vi "Array2GrayPic.vi"(7 "Pic Reference":refnum<vi>, 8 "Threshold (min)":dbl, 9 "Threshold (max)":dbl, 10 "Auto Scale?":bool, 11 "Intensity":dbl[][](array[numeric])) -> (3 "Gray Picture":picture caption="HSV to RGB Picture")   [LabVIEW 2015]
uses:
  <vilib>/picture/picture.llb/Draw True-Color Pixmap.vi
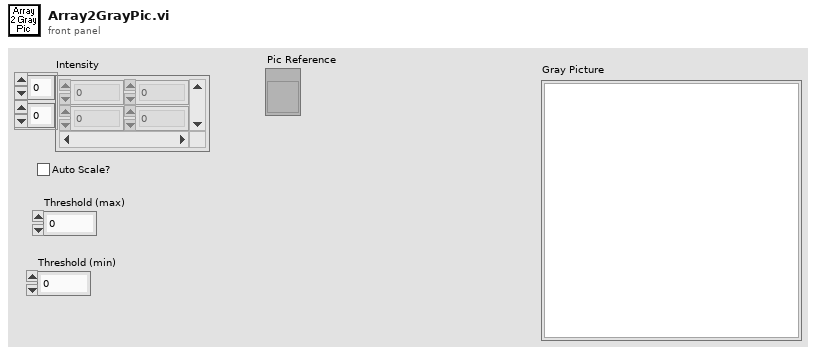
[diagram p1: front panel]
types:
  T1 = typedef "LVBoundsTypeDef.ctl" = cluster{"Width":u32, "Height":u32}
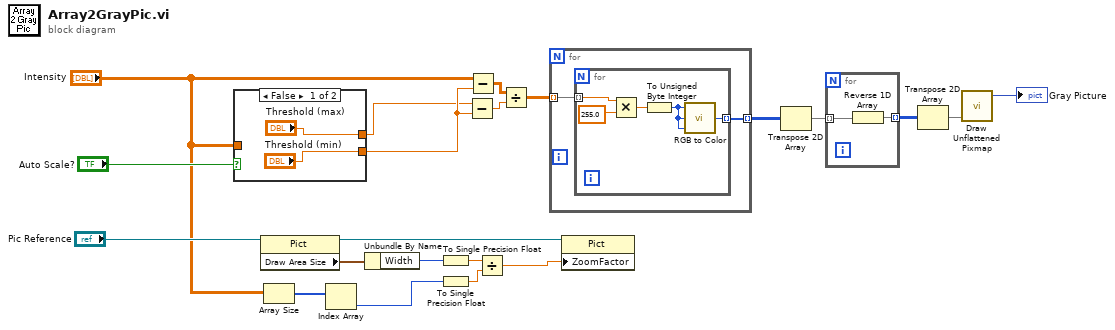
[diagram p0: block diagram]
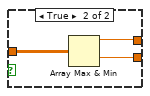
[diagram p2: hidden frame]
diagram:
  n1 = case shown="False" "Auto Scale?" {
    tunnel: "Intensity" -> [_ w26]
    tunnel: ["Threshold (max)" w25] -> w17
    tunnel: ["Threshold (min)" w24] -> w18
    frame False {
    }
    frame True {
      n2 = Array Max & Min(array=w26) -> (max value=w25:dbl, min value=w24:dbl)  [unwired: 2 out]
    }
  }
  n3 = property on="Property Node" class="Pict"(reference="Pic Reference") -> (reference out=w4:refnum<vi>, "Draw Area Size"=w6:T1)  [unwired: 1 in, 1 out]
  n4 = Array Size(array="Intensity") -> (size(s)=w2:i32[])
  n5 = Index Array(array=w2) -> (element=w1:i32)  [unwired: 1 in]
  n6 = Unbundle By Name(w6) -> ("Width"=w10:u32)
  n7 = To Single Precision Float(number=w10) -> (single precision float=w8:sgl)
  n8 = To Single Precision Float(number=w1) -> (single precision float=w9:sgl)
  n9 = Subtract(x=w17, y=w18) -> (x-y=w21:dbl)
  n10 = Subtract(x="Intensity", y=w18) -> (x-y=w20:dbl[][])
  n11 = Divide(x=w8, y=w9) -> (x/y=w5:sgl)
  n12 = Divide(x=w20, y=w21) -> (x/y=w16:dbl[][])
  n13 = for {
    tunnel: w16 -> [w28] mode=indexing
    tunnel: [w27] -> w11 mode=indexing
    n14 = for {
      tunnel: w28 -> [w30] mode=indexing
      tunnel: [w33] -> w27 mode=indexing
      n15 = Multiply(x=w30, y=255.0) -> (x*y=w31:dbl)
      n16 = To Unsigned Byte Integer(number=w31) -> (unsigned 8bit integer=w29:u8)
      n17 = call <vilib>:"RGB to Color.vi"("B"=w29, "G"=w29, "R"=w29) -> ("Color"=w33:u32)
    }
  }
  n18 = property on="Property Node" class="Pict"(reference=w4, "ZoomFactor"=w5) -> ()  [unwired: 1 in, 2 out]
  n19 = Transpose 2D Array(2D array=w11) -> (transposed array=w14:u32[][])
  n20 = for {
    tunnel: w14 -> [w35] mode=indexing
    tunnel: [w34] -> w13 mode=indexing
    n21 = Reverse 1D Array(array=w35) -> (reversed array=w34:u32[])
  }
  n22 = Transpose 2D Array(2D array=w13) -> (transposed array=w12:u32[][])
  n23 = call-poly <vilib>:"Draw Unflattened Pixmap.vi"("data (RGB format)"=w12) -> ("new picture"=→"Gray Picture":picture)  [unwired: 8 in]
